vi "Determine Shortcut Menu.vi"(8 "error in (no error)":errorcluster, 9 "SymbolIndex":T1, 10 "Menu Refnum":refnum<k9>, 11 "BrowerShortcut in":refnum<class "BrowerShortcut.lvclass">) -> (0 "error out":errorcluster, 3 "BrowerShortcut out":refnum<class "BrowerShortcut.lvclass">)   [LabVIEW 2015, in "BrowerShortcut.lvclass"]
uses:
  BrowerShortcut.lvclass
  BrowerTree/Type Definition/Symbol Index.ctl
  BrowerTree/BrowerTree.lvclass
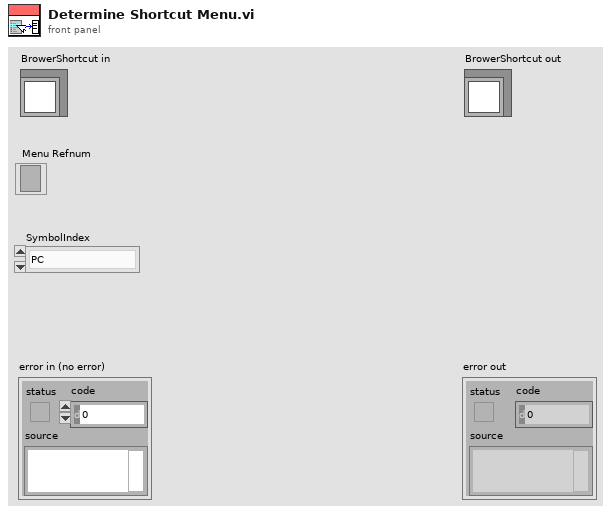
[diagram p1: front panel]
types:
  T1 = typedef "BrowerTree.lvclass/Symbol Index.ctl" = enum16{"PC", "Project", "Module", "DebugTask", "Communication"}
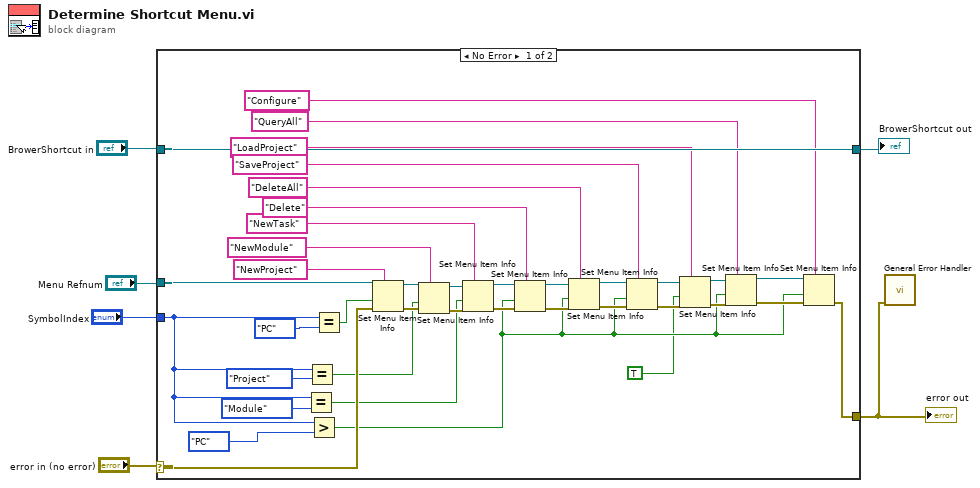
[diagram p0: block diagram]
diagram:
  n1 = case shown="No Error" "error in (no error)" {
    selector: "error in (no error)" -> [w35 w47]
    tunnel: [w19 w47] -> w1
    tunnel: [w38 w46] -> w5
    tunnel: "BrowerShortcut in" -> [w38 w46]
    tunnel: "Menu Refnum" -> [w36 _]
    tunnel: "SymbolIndex" -> [w10 _]
    frame No Error {
      n2 = Equal?(x=w10, y=Symbol_Index."Module") -> (x = y?=w7:bool)
      n3 = Equal?(x=w10, y=Symbol_Index."Project") -> (x = y?=w8:bool)
      n4 = Greater?(x=w10, y=Symbol_Index."PC") -> (0:w22:bool)
      n5 = Equal?(x=w10, y=Symbol_Index."PC") -> (x = y?=w37:bool)
      n6 = Set Menu Item Info(7:"NewProject" ("item tag"), 8:w35, 9:w37, 11:w36) -> (0:w13:errorcluster, 3:w14:refnum<k9>)  [unwired: 3 in]
      n7 = Set Menu Item Info(7:"NewModule" ("item tag"), 8:w13, 9:w8, 11:w14) -> (0:w16:errorcluster, 3:w15:refnum<k9>)  [unwired: 3 in]
      n8 = Set Menu Item Info(7:"NewTask" ("item tag"), 8:w16, 9:w7, 11:w15) -> (0:w45:errorcluster, 3:w44:refnum<k9>)  [unwired: 3 in]
      n9 = Set Menu Item Info(7:"Delete" ("item tag"), 8:w45, 9:w22, 11:w44) -> (0:w43:errorcluster, 3:w42:refnum<k9>)  [unwired: 3 in]
      n10 = Set Menu Item Info(7:"DeleteAll" ("item tag"), 8:w43, 9:w22, 11:w42) -> (0:w33:errorcluster, 3:w34:refnum<k9>)  [unwired: 3 in]
      n11 = Set Menu Item Info(7:"SaveProject" ("item tag"), 8:w33, 9:w22, 11:w34) -> (0:w30:errorcluster, 3:w31:refnum<k9>)  [unwired: 3 in]
      n12 = Set Menu Item Info(7:"LoadProject" ("item tag"), 8:w30, 9:TRUE ("enabled"), 11:w31) -> (0:w28:errorcluster, 3:w27:refnum<k9>)  [unwired: 3 in]
      n13 = Set Menu Item Info(7:"QueryAll" ("item tag"), 8:w28, 9:w22, 11:w27) -> (0:w25:errorcluster, 3:w24:refnum<k9>)  [unwired: 3 in]
      n14 = Set Menu Item Info(7:"Configure" ("item tag"), 8:w25, 9:w22, 11:w24) -> (0:w19:errorcluster)  [unwired: 3 in, 1 out]
    }
    frame Error {
    }
  }
  "error out" <- w1
  "BrowerShortcut out" <- w5
  n15 = call <vilib>:"General Error Handler.vi"("error in (no error)"=w1) -> ()  [unwired: 10 in, 5 out]
